vi "Const Configuration File Path.vi"() -> (3 "Config File Path":path)   [LabVIEW 2018, in "LF2R IDE.lvlib" / "LF2R IDE.lvclass"]
uses:
  LF2R IDE.lvclass
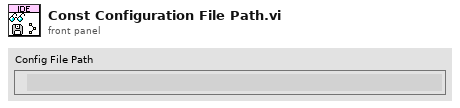
[diagram p1: front panel]
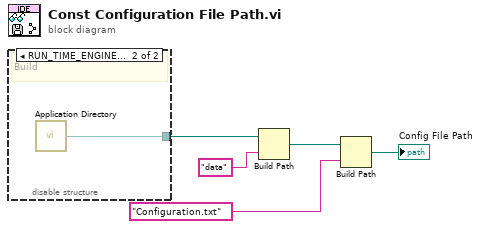
[diagram p0: block diagram]
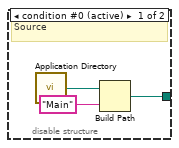
[diagram p2: hidden frame]
diagram:
  n1 = disable-structure shown="RUN_TIME_ENGINE==True" {
    disable-tunnel: [w6 w9] -> w5
    frame condition #0 (active) {
      # "Source"
      n2 = call <vilib>:"Application Directory.vi"() -> ("Application Directory"=w8:path)
      n3 = Build Path(base path=w8, name or relative path="Main") -> (appended path=w6:path)
    }
    frame condition #1 {
      # "Build"
      n4 = call <vilib>:"Application Directory.vi"() -> ("Application Directory"=w9:path)
    }
  }
  n5 = Build Path(base path=w5, name or relative path="data") -> (appended path=w3:path)
  n6 = Build Path(base path=w3, name or relative path="Configuration.txt") -> (appended path=→"Config File Path":path)
